vi "AD5781WriteRead.vi"(8 "Write":u32 format="%032b") -> (0 "WriteEqualsRead":bool, 2 "Readback 0":u32 format="%032b", 3 "Readback":u32 format="%032b")   [LabVIEW 2014]
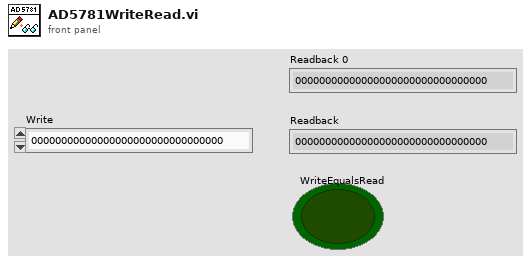
[diagram p1: front panel]
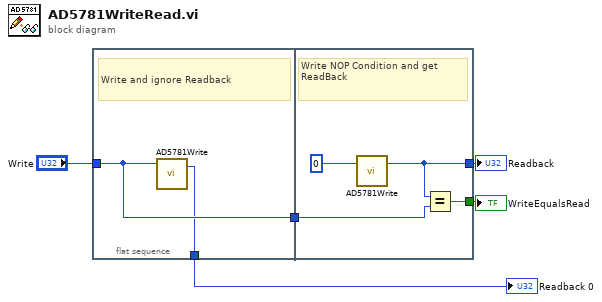
[diagram p0: block diagram]
diagram:
  n1 = flat-sequence {
    tunnel: "Write" -> [w7]
    tunnel: [w7] -> w3
    tunnel: [w6] -> w1
    tunnel: [w10] -> w4
    tunnel: w3 -> [w9]
    tunnel: [w8] -> w2
    frame #0 {
      # "Write and ignore Readback"
      n2 = call "AD5781Write.vi"("U32"=w7) -> ("Readback"=w6:u32)  [unwired: 3 in]
    }
    frame #1 {
      # "Write NOP Condition and get ReadBack"
      n3 = call "AD5781Write.vi"("U32"=u32 0) -> ("Readback"=w10:u32)  [unwired: 3 in]
      n4 = Equal?(x=w10, y=w9) -> (x = y?=w8:bool)
    }
  }
  "Readback" <- w4
  "WriteEqualsRead" <- w2
  "Readback 0" <- w1
